vi "R4Initialize.vi"(8 "error in (no error)":errorcluster) -> (0 "error out":errorcluster)   [LabVIEW 2016]
uses:
  R4SBR_SetParams.ctl
  Controls/pH_SetParams Standard.ctl
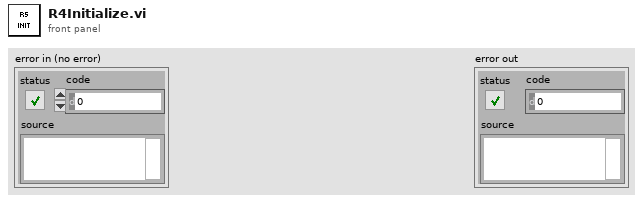
[diagram p1: front panel]
types:
  T1 = cluster{"Media Pump":bool, "Water Pump":bool, "Effluent Pump":bool, "Release Valve":bool, "Gas Pump":bool}
  T2 = cluster{"Set Point, mg/L":dbl, "Tolerance, mg/L":dbl, "N2 Valve Gain":dbl, "Air Valve Gain":dbl}
  T3 = typedef "pH_SetParams Standard.ctl" = cluster{"Set Point":dbl, "Tolerance":dbl, "Pump Time On, secs":dbl}
  T4 = typedef "R4SBR_SetParams.ctl" = cluster{"Phase":string, "Time, min":dbl, "SBR_Manual (Standard)":cluster{"Media Pump":bool, "Water Pump":bool, "Gas Pump":bool, "Effluent Pump":bool, "Release Valve":bool}}[]
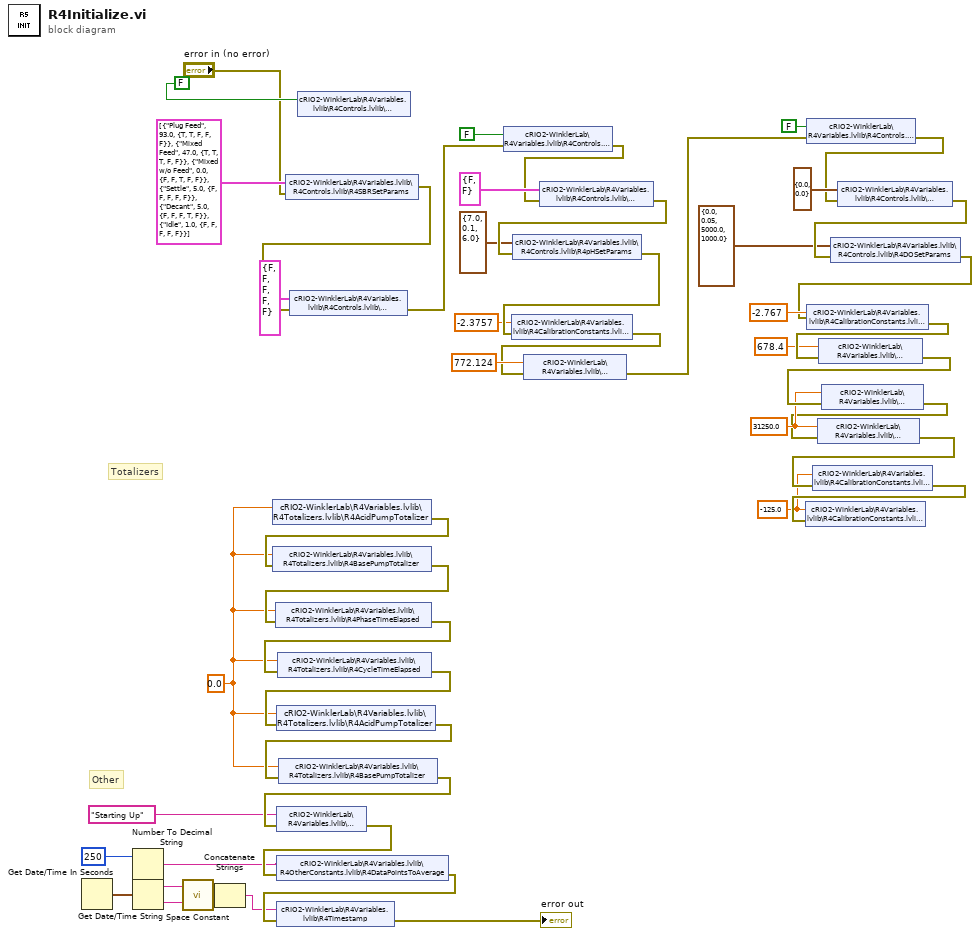
[diagram p0: block diagram]
diagram:
  w9 = 0.0 ("R1PhaseTimeElapsed")
  w19 = 31250.0 ("R1AirSlope")
  w15 = -125.0 ("R1N2Intercept")
  # "Totalizers"
  # "Other"
  n1 = Get Date/Time In Seconds() -> (seconds since 1Jan1904=w48:timestamp)
  n2 = Number To Decimal String(number=250 ("R1DataPointsToAverage")) -> (decimal integer string=w3:string)  [unwired: 1 in]
  n3 = Get Date/Time String(seconds (now)=w48) -> (date string=w45:string, time string=w47:string)  [unwired: 2 in]
  n4 = call <vilib>:"Space Constant.vi"() -> ("String"=w46:string)
  n5 = Concatenate Strings(w45, w46, w47) -> (w2:string)
  n6 = shared-variable "cRIO2-WinklerLab\\R4Variables.lvlib\\R4Totalizers.lvlib\\R4AcidPumpTotalizer"(w9) -> (error out=w14:errorcluster)  [unwired: 1 in]
  n7 = shared-variable "cRIO2-WinklerLab\\R4Variables.lvlib\\R4Totalizers.lvlib\\R4BasePumpTotalizer"(w9, error in=w14) -> (error out=w13:errorcluster)
  n8 = shared-variable "cRIO2-WinklerLab\\R4Variables.lvlib\\R4Totalizers.lvlib\\R4PhaseTimeElapsed"(w9, error in=w13) -> (error out=w12:errorcluster)
  n9 = shared-variable "cRIO2-WinklerLab\\R4Variables.lvlib\\R4Totalizers.lvlib\\R4CycleTimeElapsed"(w9, error in=w12) -> (error out=w11:errorcluster)
  n10 = shared-variable "cRIO2-WinklerLab\\R4Variables.lvlib\\R4Totalizers.lvlib\\R4AcidPumpTotalizer"(w9, error in=w11) -> (error out=w10:errorcluster)
  n11 = shared-variable "cRIO2-WinklerLab\\R4Variables.lvlib\\R4Totalizers.lvlib\\R4BasePumpTotalizer"(w9, error in=w10) -> (error out=w8:errorcluster)
  n12 = shared-variable "cRIO2-WinklerLab\\R4Variables.lvlib\\R4Status"("Starting Up" ("R1Status"), error in=w8) -> (error out=w7:errorcluster)
  n13 = shared-variable "cRIO2-WinklerLab\\R4Variables.lvlib\\R4OtherConstants.lvlib\\R4DataPointsToAverage"(w3, error in=w7) -> (error out=w5:errorcluster)
  n14 = shared-variable "cRIO2-WinklerLab\\R4Variables.lvlib\\R4Timestamp"(w2, error in=w5) -> (error out=→"error out":errorcluster)
  n15 = shared-variable "cRIO2-WinklerLab\\R4Variables.lvlib\\R4Controls.lvlib\\R4SBRSetParams"(T4 [{"Phase"="Plug Feed", "Time, min"=93.0, "SBR_Manual (Standard)"={"Media Pump"=TRUE, "Water Pump"=TRUE, "Gas Pump"=FALSE, "Effluent Pump"=FALSE, "Release Valve"=FALSE}}, {"Phase"="Mixed Feed", "Time, min"=47.0, "SBR_Manual (Standard)"={"Media Pump"=TRUE, "Water Pump"=TRUE, "Gas Pump"=TRUE, "Effluent Pump"=FALSE, "Release Valve"=FALSE}}, {"Phase"="Mixed w/o Feed", "Time, min"=0.0, "SBR_Manual (Standard)"={"Media Pump"=FALSE, "Water Pump"=FALSE, "Gas Pump"=TRUE, "Effluent Pump"=FALSE, "Release Valve"=FALSE}}, {"Phase"="Settle", "Time, min"=5.0, "SBR_Manual (Standard)"={"Media Pump"=FALSE, "Water Pump"=FALSE, "Gas Pump"=FALSE, "Effluent Pump"=FALSE, "Release Valve"=FALSE}}, {"Phase"="Decant", "Time, min"=5.0, "SBR_Manual (Standard)"={"Media Pump"=FALSE, "Water Pump"=FALSE, "Gas Pump"=FALSE, "Effluent Pump"=TRUE, "Release Valve"=FALSE}}, {"Phase"="Idle", "Time, min"=1.0, "SBR_Manual (Standard)"={"Media Pump"=FALSE, "Water Pump"=FALSE, "Gas Pump"=FALSE, "Effluent Pump"=FALSE, "Release Valve"=FALSE}}] ("R1SBR_SetParams 2"), error in="error in (no error)") -> (error out=w41:errorcluster)
  n16 = shared-variable "cRIO2-WinklerLab\\R4Variables.lvlib\\R4Controls.lvlib\\R4SBRManual"(T1 {"Media Pump"=FALSE, "Water Pump"=FALSE, "Effluent Pump"=FALSE, "Release Valve"=FALSE, "Gas Pump"=FALSE} ("R4SBRManual"), error in=w41) -> (error out=w39:errorcluster)
  n17 = shared-variable "cRIO2-WinklerLab\\R4Variables.lvlib\\R4Controls.lvlib\\R4SBRSwitch"(FALSE ("R1SBRSwitch")) -> ()  [unwired: 1 in, 1 out]
  n18 = shared-variable "cRIO2-WinklerLab\\R4Variables.lvlib\\R4Controls.lvlib\\R4pHSwitch"(FALSE ("R1pHSwitch"), error in=w39) -> (error out=w37:errorcluster)
  n19 = shared-variable "cRIO2-WinklerLab\\R4Variables.lvlib\\R4Controls.lvlib\\R4pHManual"(cluster{"Acid Pump":bool, "Base Pump":bool} {"Acid Pump"=FALSE, "Base Pump"=FALSE} ("R1pHManual"), error in=w37) -> (error out=w36:errorcluster)
  n20 = shared-variable "cRIO2-WinklerLab\\R4Variables.lvlib\\R4Controls.lvlib\\R4pHSetParams"(T3 {"Set Point"=7.0, "Tolerance"=0.1, "Pump Time On, secs"=6.0} ("R1pHSetParams"), error in=w36) -> (error out=w34:errorcluster)
  n21 = shared-variable "cRIO2-WinklerLab\\R4Variables.lvlib\\R4CalibrationConstants.lvlib\\R4pHIntercept"(-2.3757 ("R12pHInt"), error in=w34) -> (error out=w31:errorcluster)
  n22 = shared-variable "cRIO2-WinklerLab\\R4Variables.lvlib\\R4CalibrationConstants.lvlib\\R4pHSlope"(772.124 ("R1pHSlope"), error in=w31) -> (error out=w29:errorcluster)
  n23 = shared-variable "cRIO2-WinklerLab\\R4Variables.lvlib\\R4Controls.lvlib\\R4pHSwitch"(FALSE ("R1pHSwitch"), error in=w29) -> (error out=w27:errorcluster)
  n24 = shared-variable "cRIO2-WinklerLab\\R4Variables.lvlib\\R4Controls.lvlib\\R4DOManual"(cluster{"Air MFC":dbl, "N2 MFC":dbl} {"Air MFC"=0.0, "N2 MFC"=0.0} ("R1DOManual"), error in=w27) -> (error out=w26:errorcluster)
  n25 = shared-variable "cRIO2-WinklerLab\\R4Variables.lvlib\\R4Controls.lvlib\\R4DOSetParams"(T2 {"Set Point, mg/L"=0.0, "Tolerance, mg/L"=0.05, "N2 Valve Gain"=5000.0, "Air Valve Gain"=1000.0} ("R1DOSetParams"), error in=w26) -> (error out=w23:errorcluster)
  n26 = shared-variable "cRIO2-WinklerLab\\R4Variables.lvlib\\R4CalibrationConstants.lvlib\\R4DOIntercept"(-2.767 ("R1DOInt"), error in=w23) -> (error out=w22:errorcluster)
  n27 = shared-variable "cRIO2-WinklerLab\\R4Variables.lvlib\\R4CalibrationConstants.lvlib\\R4DOSlope"(678.4 ("R1DOSlope"), error in=w22) -> (error out=w20:errorcluster)
  n28 = shared-variable "cRIO2-WinklerLab\\R4Variables.lvlib\\R4CalibrationConstants.lvlib\\R4N2Slope"(w19, error in=w20) -> (error out=w18:errorcluster)
  n29 = shared-variable "cRIO2-WinklerLab\\R4Variables.lvlib\\R4CalibrationConstants.lvlib\\R4AirSlope"(w19, error in=w18) -> (error out=w17:errorcluster)
  n30 = shared-variable "cRIO2-WinklerLab\\R4Variables.lvlib\\R4CalibrationConstants.lvlib\\R4AirIntercept"(w15, error in=w17) -> (error out=w16:errorcluster)
  n31 = shared-variable "cRIO2-WinklerLab\\R4Variables.lvlib\\R4CalibrationConstants.lvlib\\R4N2Intercept"(w15, error in=w16) -> ()  [unwired: 1 out]
